vi "Bumber to Button.vi"(2 "Bumber / Axis 2":dbl, 3 "Bumber / Axis":dbl) -> (0 "Output 2":bool, 1 "Output":bool)   [LabVIEW 2017]
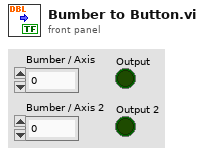
[diagram p1: front panel]
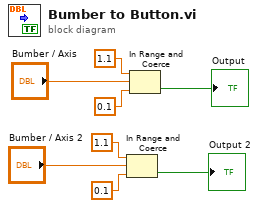
[diagram p0: block diagram]
diagram:
  n1 = In Range and Coerce(upper limit=1.1, x="Bumber / Axis 2", lower limit=0.1) -> (In Range?=→"Output 2":bool)  [unwired: 1 out]
  n2 = In Range and Coerce(upper limit=1.1, x="Bumber / Axis", lower limit=0.1) -> (In Range?=→"Output":bool)  [unwired: 1 out]
